vi "SwrvLinAlg Full Spin Logic.vi"(8 "E>A Floor":dbl, 9 "Drive Wheel":dbl, 10 "Target Angle":dbl, 11 "Current Encoder Angle":dbl) -> (0 "Wheel Reversed":bool, 1 "Position Error 360":dbl, 2 "Adjusted Drive":dbl, 3 "Spin Wheel Command":dbl, 4 "Position Error":dbl, 6 "Position Error 180":dbl)   [LabVIEW 2017]
panel:
  # "0-360 Degrees"
  # "0-360 Degrees"
  # "CTRE Encoder"
  # "PWM"
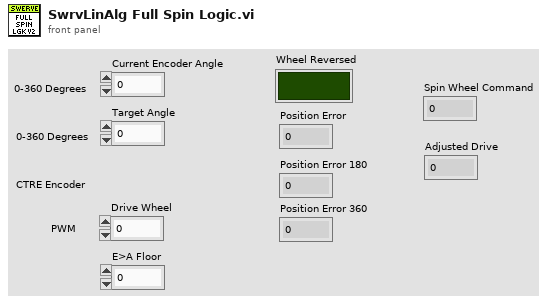
[diagram p1: front panel]
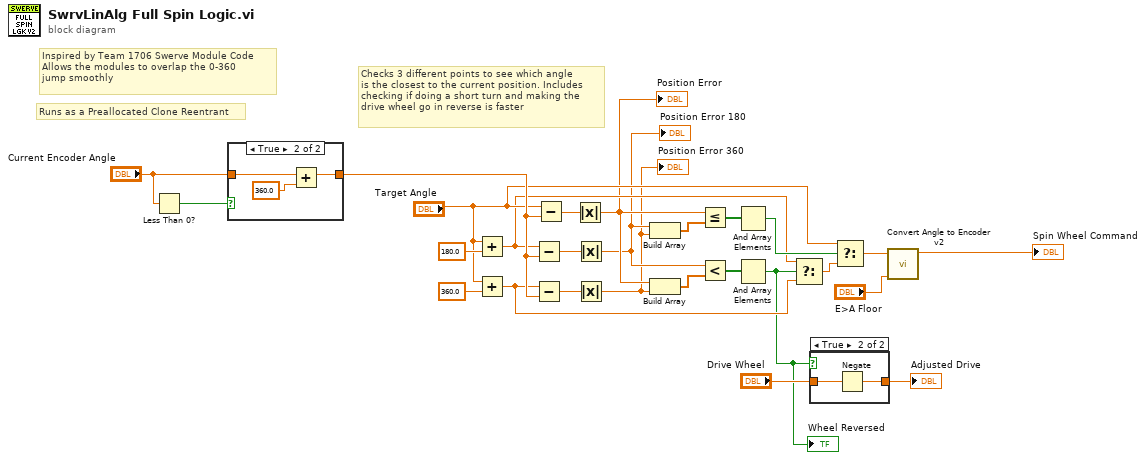
[diagram p0: block diagram]
diagram:
  # "Runs as a Preallocated Clone Reentrant"
  # "Checks 3 different points to see which angle\nis the closest to the current position. Includes\nchecking if doing a short turn and making the\ndrive wheel go in reverse is faster"
  # "Inspired by Team 1706 Swerve Module Code\nAllows the modules to overlap the 0-360 \njump smoothly"
  n1 = Less Than 0?(x="Current Encoder Angle") -> (x < 0?=w2:bool)
  n2 = case shown="True" w2 {
    tunnel: "Current Encoder Angle" -> [w27 w29]
    tunnel: [w27 w28] -> w23
    frame False {
    }
    frame True {
      n3 = Add(x=w29, y=360.0) -> (x+y=w28:dbl)
    }
  }
  n4 = Add(x="Target Angle", y=180.0) -> (x+y=w11:dbl)
  n5 = Add(x="Target Angle", y=360.0) -> (x+y=w10:dbl)
  n6 = Subtract(x=w11, y=w23) -> (x-y=w15:dbl)
  n7 = Subtract(x=w10, y=w23) -> (x-y=w16:dbl)
  n8 = Subtract(x="Target Angle", y=w23) -> (x-y=w14:dbl)
  n9 = Absolute Value(x=w14) -> (abs(x)=w6:dbl)
  "Position Error" <- w6
  n10 = Absolute Value(x=w15) -> (abs(x)=w5:dbl)
  "Position Error 180" <- w5
  n11 = Absolute Value(x=w16) -> (abs(x)=w4:dbl)
  "Position Error 360" <- w4
  n12 = Build Array(w5, w4) -> (w22:dbl[])
  n13 = Build Array(w6, w4) -> (w20:dbl[])
  n14 = Less Or Equal?(x=w6, y=w22) -> (x <= y?=w21:bool[])
  n15 = Less?(x=w5, y=w20) -> (x < y?=w19:bool[])
  n16 = And Array Elements(Boolean array=w21) -> (logical AND=w17:bool)
  n17 = And Array Elements(Boolean array=w19) -> (logical AND=w7:bool)
  "Wheel Reversed" <- w7
  n18 = Select(t=w11, s=w7, f=w10) -> (s? t:f=w18:dbl)
  n19 = case shown="True" w7 {
    tunnel: [w31 w33] -> w9
    tunnel: "Drive Wheel" -> [w31 w32]
    frame False {
    }
    frame True {
      n20 = Negate(x=w32) -> (-x=w33:dbl)
    }
  }
  "Adjusted Drive" <- w9
  n21 = Select(t="Target Angle", s=w17, f=w18) -> (s? t:f=w13:dbl)
  n22 = call "Convert Angle to Encoder v2.vi"("Floor"="E>A Floor", "Angle"=w13) -> ("Encoder Units"=→"Spin Wheel Command":dbl)  [unwired: 9 in]
